vi "IMAQdx_getAttribute_Enum.vi"(3 "error in (no error)":errorcluster, 4 "Attribute Name":string, 5 "IMAQdx Session":T1) -> (0 "error out":errorcluster, 1 "IMAQdx Attribute":variant, 2 "dup IMAQdx Session":T1)   [LabVIEW 2014, in "HGF_VisionTools.lvlib"]
doc: "This VI reads IMAQdx attribute value of type enumeration and its properties. Value is returned as Variant and properties as Variant attributes."
uses:
  HGF_VisionTools.lvlib
  <resource>/objmgr/imaqdx.rc
  <vilib>/userdefined/High Color/IMAQdx.ctl
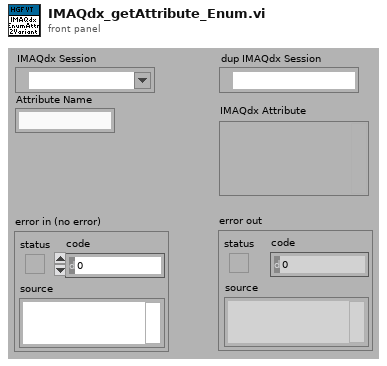
[diagram p1: front panel]
types:
  T1 = typedef "IMAQdx.ctl" = refnum<k21>
  T2 = cluster{"EnumStrings[]":void, "EnumValues[]":void}
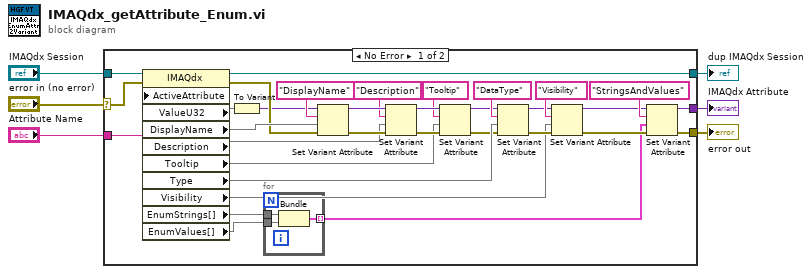
[diagram p0: block diagram]
diagram:
  n1 = case shown="No Error" "error in (no error)" {
    selector: "error in (no error)" -> [w7 w43]
    tunnel: "IMAQdx Session" -> [w39 w44]
    tunnel: "Attribute Name" -> [w38 _]
    tunnel: [w37 w44] -> w4
    tunnel: [w9 w43] -> w3
    tunnel: [w8 _] -> w2
    frame No Error {
      n2 = property class="IMAQdx"(reference=w39, error in=w7, "ActiveAttribute"=w38) -> (reference out=w37:T1, error out=w34:errorcluster, "ValueU32"=w33, "DisplayName"=w35, "Description"=w23, "Tooltip"=w22, "Type"=w21, "Visibility"=w17, "EnumStrings[]"=w12, "EnumValues[]"=w11)
      n3 = To Variant(anything=w33) -> (Variant=w32:variant)
      n4 = for {
        tunnel: w12 -> [w42]
        tunnel: w11 -> [w41]
        tunnel: [w40] -> w10 mode=indexing
        n5 = Bundle("EnumStrings[]"=w42, "EnumValues[]"=w41) -> (w40:T2)  [unwired: 1 in]
      }
      n6 = Set Variant Attribute(Variant=w32, name="DisplayName", value=w35, error in=w34) -> (Variant out=w31:variant, error out=w28:errorcluster)  [unwired: 1 out]
      n7 = Set Variant Attribute(Variant=w31, name="Description", value=w23, error in=w28) -> (Variant out=w30:variant, error out=w29:errorcluster)  [unwired: 1 out]
      n8 = Set Variant Attribute(Variant=w30, name="Tooltip", value=w22, error in=w29) -> (Variant out=w16:variant, error out=w15:errorcluster)  [unwired: 1 out]
      n9 = Set Variant Attribute(Variant=w16, name="DataType", value=w21, error in=w15) -> (Variant out=w18:variant, error out=w19:errorcluster)  [unwired: 1 out]
      n10 = Set Variant Attribute(Variant=w18, name="Visibility", value=w17, error in=w19) -> (Variant out=w14:variant, error out=w13:errorcluster)  [unwired: 1 out]
      n11 = Set Variant Attribute(Variant=w14, name="StringsAndValues", value=w10, error in=w13) -> (Variant out=w8:variant, error out=w9:errorcluster)  [unwired: 1 out]
    }
    frame Error {
    }
  }
  "IMAQdx Attribute" <- w2
  "dup IMAQdx Session" <- w4
  "error out" <- w3
